vi "Create All Message Queues.vi"(8 "error in (no error)":errorcluster) -> (0 "error out":errorcluster, 3 "Message Queues out":T1)   [LabVIEW 2014]
uses:
  Controls/Message Cluster.ctl
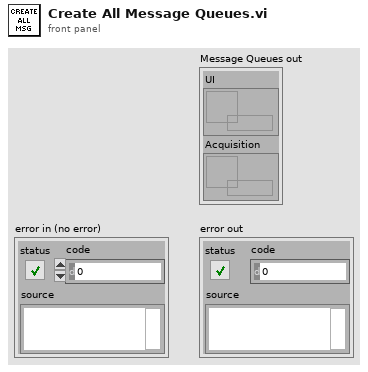
[diagram p1: front panel]
types:
  T1 = cluster{"UI":refnum<queue>, "Acquisition":refnum<queue>}
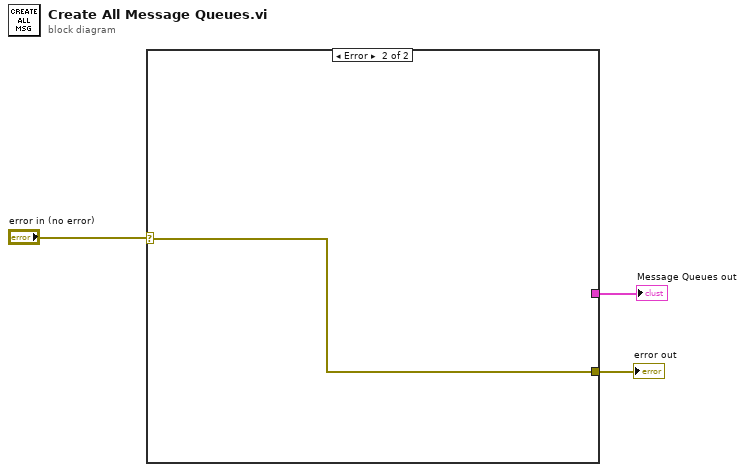
[diagram p0: block diagram]
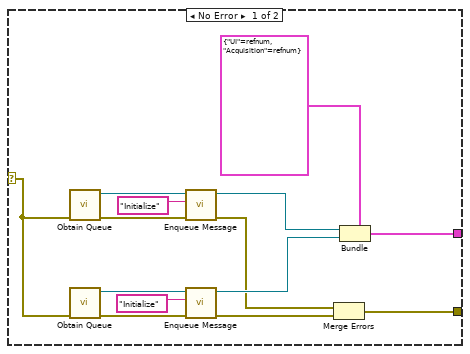
[diagram p2: hidden frame]
diagram:
  n1 = case shown="Error" "error in (no error)" {
    selector: "error in (no error)" -> [w17 w18]
    tunnel: [w5 w18] -> w2
    tunnel: [w4 _] -> w3
    frame No Error {
      n2 = call "Obtain Queue.vi"("error in (no error)"=w17) -> ("error out"=w13:errorcluster, "Queue out"=w16:refnum<queue>)  [unwired: 9 in]
      n3 = call "Obtain Queue.vi"("error in (no error)"=w17) -> ("error out"=w14:errorcluster, "Queue out"=w15:refnum<queue>)  [unwired: 9 in]
      n4 = call "Enqueue Message.vi"("error in (no error)"=w13, "Message"="Initialize", "Queue in"=w16) -> ("error out"=w6:errorcluster, "Queue out"=w9:refnum<queue>)  [unwired: 7 in]
      n5 = call "Enqueue Message.vi"("error in (no error)"=w14, "Message"="Initialize", "Queue in"=w15) -> ("error out"=w7:errorcluster, "Queue out"=w8:refnum<queue>)  [unwired: 7 in]
      n6 = Merge Errors(w6, w7) -> (w5:errorcluster)
      n7 = Bundle(cluster=T1 {"UI"=refnum, "Acquisition"=refnum}, "UI"=w9, "Acquisition"=w8) -> (w4:T1)
    }
    frame Error {
    }
  }
  "Message Queues out" <- w3
  "error out" <- w2
